vi "RequestJSONTest.vi"() -> (0 "error out":errorcluster, 2 "Pass":bool)   [LabVIEW 2015]
uses:
  Request/RequestType.ctl
  Request/PersonnelType.ctl
  Request/Request.lvclass/Request.ctl
  Request/Write AckName.vi
  Request/Write AckTime.vi
  Request/Write FulfilledTime.vi
  Request/Write FulfilledName.vi
  Request/Read AckName.vi
  Request/Read AckTime.vi
  Request/Read Alarm.vi
  Request/Read Description.vi
  Request/Read FulfilledName.vi
  Request/Read FulfilledTime.vi
  Request/Read PersonnelType.vi
  Request/Read Request Type.vi
  Request/Read RequestID.vi
  Request/Read Room Number.vi
  Request/Read StartName.vi
  Request/Read StartTime.vi
  Request/Read Summary.vi
  Request/Request.lvclass
panel:
  out "Summary":bool
  out "StartTime":bool
  out "StartName":bool
  out "RoomNumber":bool
  out "Request ID":bool
  out "RequestType":bool
  out "PersonnelType":bool
  out "FullfilledTime":bool
  out "FulfilledName":bool
  out "Description":bool
  out "Alarm":bool
  out "AckTime":bool
  out "AckName":bool
  out "Request UID":string
  in  "Personnel Type":T1 items=["Nurse", "Doctor", "Cleanning", "Admin"]
  in  "Name":string
  in  "error in (no error)":errorcluster
  in  "Room Number":i32
  in  "Request Type":T2
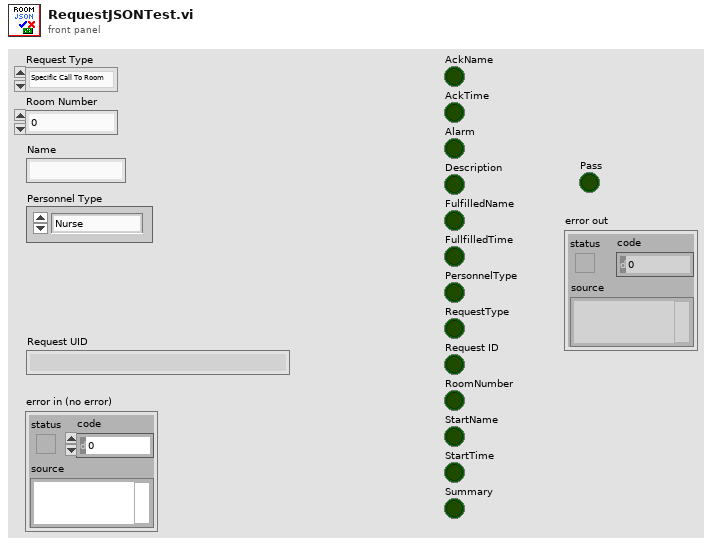
[diagram p1: front panel]
types:
  T1 = typedef "Request.lvclass/PersonnelType.ctl" = u16
  T2 = typedef "Request.lvclass/RequestType.ctl" = enum16{"Specific Call To Room", "General Call To Room"}
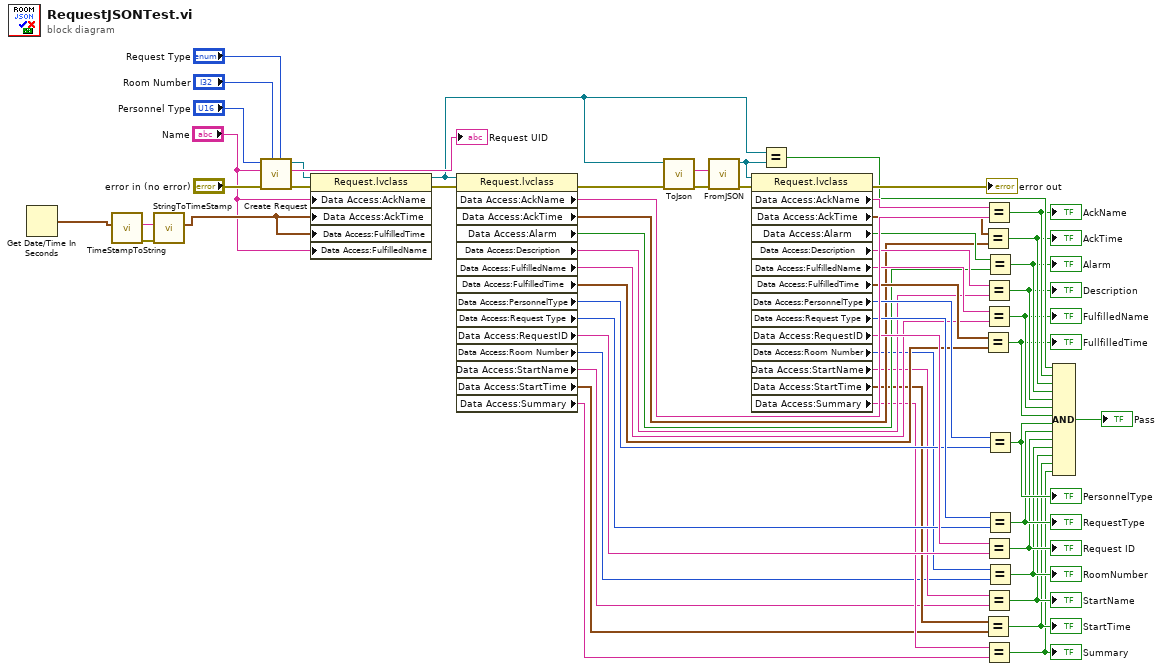
[diagram p0: block diagram]
diagram:
  n1 = Get Date/Time In Seconds() -> (seconds since 1Jan1904=w5:timestamp)
  n2 = call "TimeStampToString.vi"("Time Stamp"=w5) -> ("error out"=w3:errorcluster, "String"=w4:string)  [unwired: 9 in]
  n3 = call "StringToTimeStamp.vi"("error in (no error)"=w3, "TimeStamp"=w4) -> ("Time Stamp"=w2:timestamp)  [unwired: 8 in, 1 out]
  n4 = call "Create Request.vi"("Request Type"="Request Type", "Room Number"="Room Number", "error in (no error)"="error in (no error)", "Name"="Name", "Personnel Type"="Personnel Type") -> ("error out"=w53:errorcluster, "RUID"=→"Request UID":string, "Request out"=w7:refnum<class "Request.lvclass">)  [unwired: 4 in]
  n5 = property class="Request.lvclass"(reference=w7, error in=w53, "Data Access:AckName"="Name", "Data Access:AckTime"=w2, "Data Access:FulfilledTime"=w2, "Data Access:FulfilledName"="Name") -> (reference out=w6:refnum<class "Request.lvclass">, error out=w8:errorcluster)
  n6 = property class="Request.lvclass"(reference=w6, error in=w8) -> (error out=w52:errorcluster, "Data Access:AckName"=w49:string, "Data Access:AckTime"=w40:timestamp, "Data Access:Alarm"=w39:bool, "Data Access:Description"=w38:string, "Data Access:FulfilledName"=w37:string, "Data Access:FulfilledTime"=w36:timestamp, "Data Access:PersonnelType"=w35:T1, "Data Access:Request Type"=w34:T2, "Data Access:RequestID"=w33:string, "Data Access:Room Number"=w24:i32, "Data Access:StartName"=w25:string, "Data Access:StartTime"=w26:timestamp, "Data Access:Summary"=w27:string)  [unwired: 1 out]
  n7 = call "ToJson.vi"("error in (no error)"=w52, "Request"=w6) -> ("error out"=w51:errorcluster, "Request"=w56:string)  [unwired: 8 in]
  n8 = call "FromJSON.vi"("error in (no error)"=w51, "Request"=w56) -> ("error out"=w55:errorcluster, "Request out"=w54:refnum<class "Request.lvclass">)  [unwired: 8 in]
  n9 = property class="Request.lvclass"(reference=w54, error in=w55) -> (error out=→"error out":errorcluster, "Data Access:AckName"=w50:string, "Data Access:AckTime"=w48:timestamp, "Data Access:Alarm"=w47:bool, "Data Access:Description"=w46:string, "Data Access:FulfilledName"=w45:string, "Data Access:FulfilledTime"=w44:timestamp, "Data Access:PersonnelType"=w43:T1, "Data Access:Request Type"=w42:T2, "Data Access:RequestID"=w41:string, "Data Access:Room Number"=w31:i32, "Data Access:StartName"=w30:string, "Data Access:StartTime"=w29:timestamp, "Data Access:Summary"=w28:string)  [unwired: 1 out]
  n10 = Equal?(x=w6, y=w54) -> (x = y?=w23:bool)
  n11 = Equal?(x=w48, y=w40) -> (x = y?=w21:bool)
  "AckTime" <- w21
  n12 = Equal?(x=w44, y=w36) -> (x = y?=w17:bool)
  "FullfilledTime" <- w17
  n13 = Equal?(x=w29, y=w26) -> (x = y?=w11:bool)
  "StartTime" <- w11
  n14 = Equal?(x=w50, y=w49) -> (x = y?=w22:bool)
  "AckName" <- w22
  n15 = Equal?(x=w46, y=w38) -> (x = y?=w19:bool)
  "Description" <- w19
  n16 = Equal?(x=w45, y=w37) -> (x = y?=w18:bool)
  "FulfilledName" <- w18
  n17 = Equal?(x=w41, y=w33) -> (x = y?=w14:bool)
  "Request ID" <- w14
  n18 = Equal?(x=w30, y=w25) -> (x = y?=w12:bool)
  "StartName" <- w12
  n19 = Equal?(x=w28, y=w27) -> (x = y?=w10:bool)
  "Summary" <- w10
  n20 = Equal?(x=w47, y=w39) -> (x = y?=w20:bool)
  "Alarm" <- w20
  n21 = Equal?(x=w43, y=w35) -> (x = y?=w16:bool)
  "PersonnelType" <- w16
  n22 = Equal?(x=w42, y=w34) -> (x = y?=w15:bool)
  "RequestType" <- w15
  n23 = Equal?(x=w31, y=w24) -> (x = y?=w13:bool)
  "RoomNumber" <- w13
  n24 = Compound Arithmetic op=AND(w23, w22, w21, w20, w19, w18, w17, w16, w15, w14, w13, w12, w11, w10) -> (→"Pass":bool)
